vi "InputLimitVoltage.vi"() -> (1 "CW 2":bool, 2 "Output Limit Voltage":i16)   [LabVIEW 2016]
uses:
  user/GrobaLimitVoltage.vi
panel:
  in  "CW":bool
  in  "Boolean":bool
  in  "Input Limit Voltage(hidden)":i16=70
  in  "String":string
  in  "Change LimitVoltage":bool caption="OK"
  in  "Input Limit Voltage":i16=70
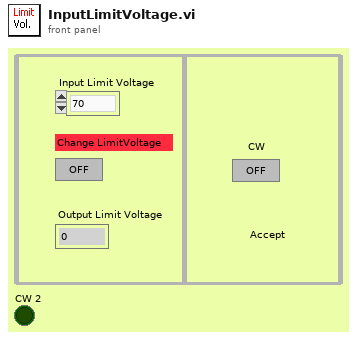
[diagram p1: front panel]
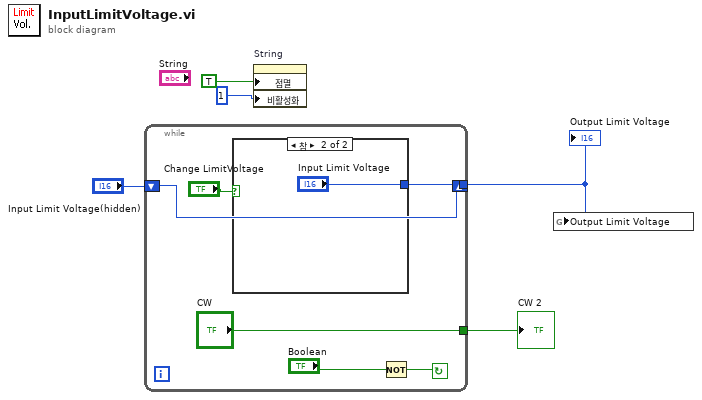
[diagram p0: block diagram]
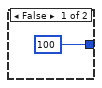
[diagram p2: hidden frame]
diagram:
  n1 = while {
    shift-right: [w9] -> _
    shift-left: "Input Limit Voltage(hidden)" -> [w9]
    tunnel: [w10] -> w2
    tunnel: ["CW"] -> w1
    stop <- w11 continue-if-true
    n2 = case shown="참" "Change LimitVoltage" {
      tunnel: [100 "Input Limit Voltage"] -> w10
      frame False {
      }
      frame True {
      }
    }
    n3 = Not(x="Boolean") -> (.not. x?=w11:bool)
  }
  "Output Limit Voltage" <- w2
  "CW 2" <- w1
  n4 = property on="String" class="Str"("점멸"=TRUE ("Write Attribute"), "비활성화"=u8 1 ("Write Attribute")) -> ()  [unwired: 2 in, 2 out]
  n5 = global write "GrobaLimitVoltage.vi" "Output Limit Voltage"(w2) -> ()
